vi "GUI_BELLA_CapStage.vi"() -> ()   [LabVIEW 2013]
uses:
  shared programs/GUI_Template/GUI_master/tcp_new_data_event.ctl
  shared programs/GUI_Template/GUI_master/tcp new data cluster.ctl
panel:
  in  "Stop":bool
  in  "position::1":enum16{"out", "in", "Unknown"}(ring) caption="POSITION"
  in  "GUIdevice 1":string="PL1-Stage-Cap"
  out "tcp data event":T1
  out "error IO 2":errorcluster
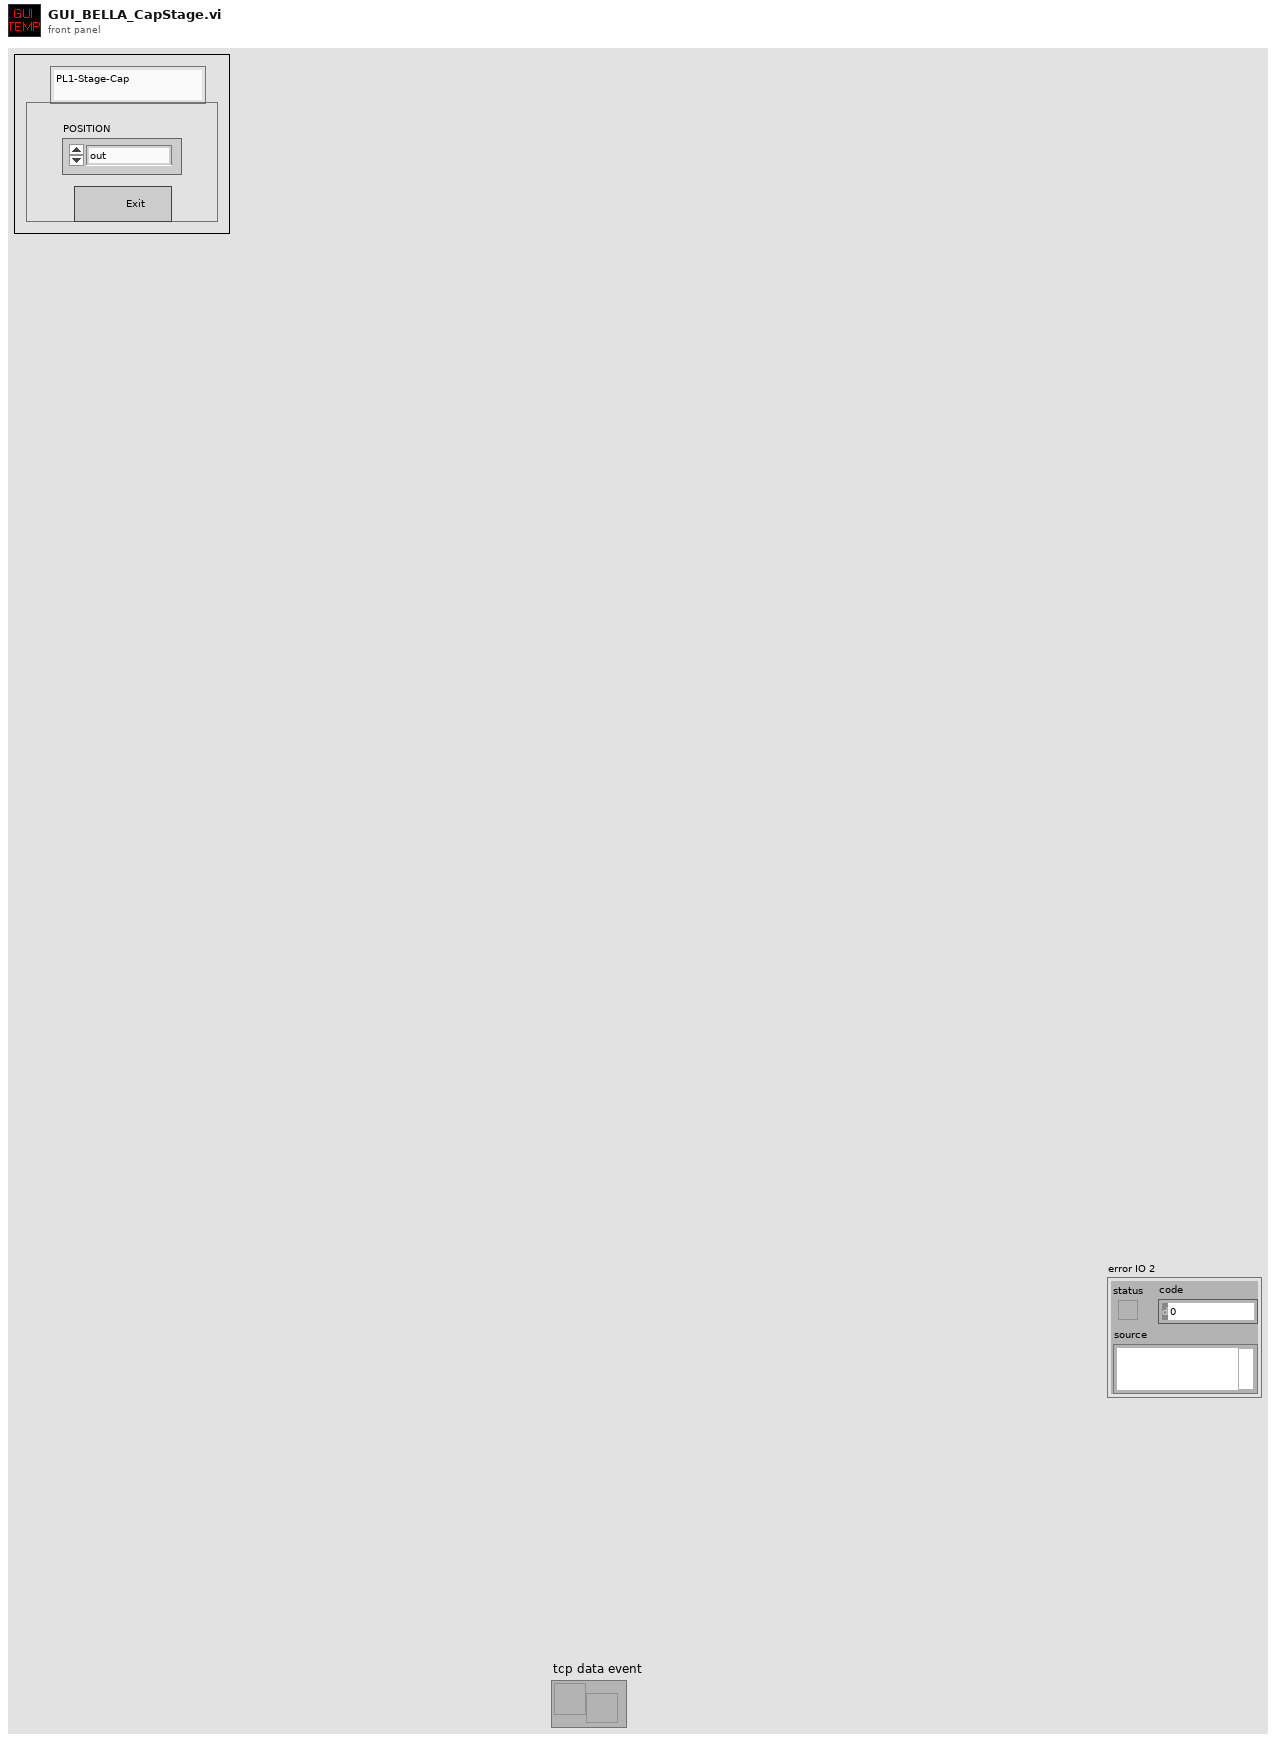
[diagram p1: front panel]
types:
  T1 = typedef "tcp_new_data_event.ctl" = refnum<user-event>
  T2 = typedef "tcp new data cluster.ctl" = cluster{"EventEnum":enum16{"new data", "connection status update"}, "Device name":string}
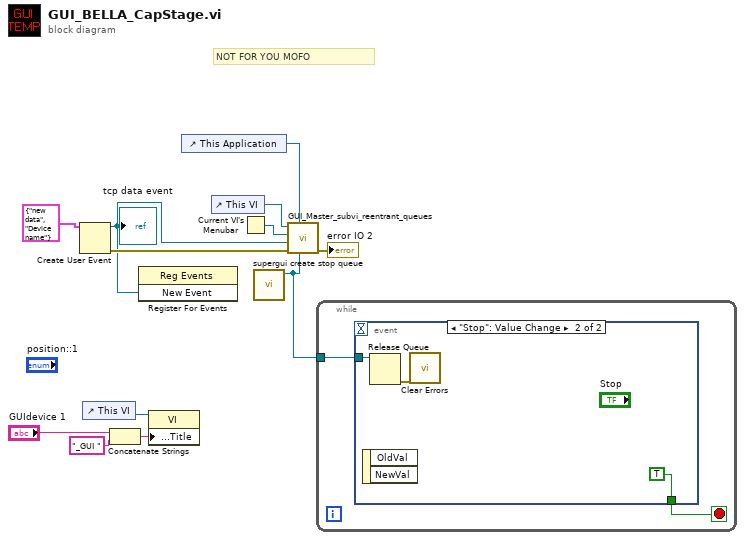
[diagram p0: block diagram]
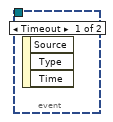
[diagram p2: hidden frame]
diagram:
  # "NOT FOR YOU MOFO"
  n1 = Create User Event(user event datatype=T2 {"EventEnum"=enum."new data", "Device name"="Device name"} ("New Event")) -> (user event=w7:refnum<user-event>, error out=w8:errorcluster)  [unwired: 1 in]
  "tcp data event" <- w7
  n2 = control-ref of="This VI"() -> (w5:refnum<vi>)
  n3 = Concatenate Strings("GUIdevice 1", "_GUI ") -> (w4:string)
  n4 = register-events(w7) -> ()  [unwired: 2 in, 2 out]
  n5 = property class="VI"(reference=w5, "Front Panel.Title"=w4) -> ()  [unwired: 1 in, 2 out]
  n6 = control-ref of="This Application"() -> (w6:refnum<vi>)
  n7 = control-ref of="This VI"() -> (w11:refnum<vi>)
  n8 = Current VI's Menubar() -> (w10:refnum<k9>)
  n9 = call "supergui create stop queue.vi"() -> ("STOP Queue out"=w1:refnum<queue>)  [unwired: 11 in]
  n10 = call "GUI_Master_subvi_reentrant_queues.vi"("STOP Queue in"=w1, "This Application"=w6, "error in (no error)"=w8, "tcp data event"=w7, "Caller menu reference"=w10, "Caller VI ref"=w11) -> ("error out"=→"error IO 2":errorcluster)  [unwired: 5 in]
  n11 = while {
    tunnel: w1 -> [w13]
    stop <- w14 stop-if-true
    n12 = event shown="[1] \"Stop\": Value Change" {
      selector: _ -> [_ _]
      dyn-events: _ -> [_ _]
      timeout: _ -> [_ _]
      tunnel: [_ TRUE] -> w14
      tunnel: w13 -> [_ w16]
      event Timeout {
        n13 = event-data() -> ()  [unwired: 1 in, 3 out]
      }
      event "Stop": Value Change {
        n14 = event-data() -> ()  [unwired: 1 in, 2 out]
        n15 = Release Queue(queue=w16) -> (error out=w15:errorcluster)  [unwired: 2 in, 2 out]
        n16 = call <vilib>:"Clear Errors.vi"("error in (no error)"=w15) -> ()  [unwired: 6 in, 1 out]
      }
    }
  }
